vi "Keithley_Output_to_Number_1_and_2.vi"(6 "GPIB = true, RS-232 = false":bool, 10 "string":string) -> (1 "number 2":dbl, 2 "number 1":dbl, 3 "array":dbl[](array[numeric]))   [LabVIEW 2018]
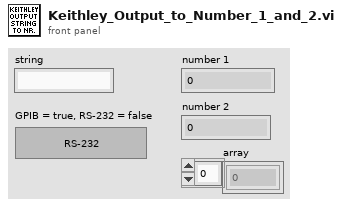
[diagram p1: front panel]
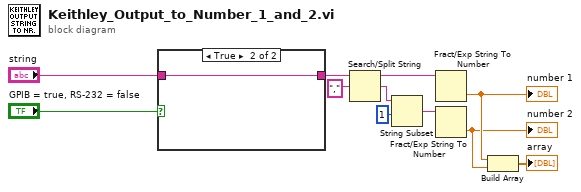
[diagram p0: block diagram]
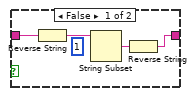
[diagram p2: hidden frame]
diagram:
  n1 = case shown="True" "GPIB = true, RS-232 = false" {
    tunnel: "string" -> [w13 w16]
    tunnel: [w12 w16] -> w2
    frame False {
      (unwired) 1
      n2 = Reverse String(1:w13) -> (0:w15:string)
      n3 = String Subset(string=w15) -> (substring=w14:string)  [unwired: 2 in]
      n4 = Reverse String(1:w14) -> (0:w12:string)
    }
    frame True {
    }
  }
  n5 = Search/Split String(string=w2, search string/char (-)=",") -> (substring before match=w7:string, match + rest of string=w10:string)  [unwired: 1 in, 1 out]
  n6 = String Subset(string=w10, offset (0)=1) -> (substring=w11:string)  [unwired: 1 in]
  n7 = Fract/Exp String To Number(string=w7) -> (number=w6:dbl)  [unwired: 3 in, 1 out]
  "number 1" <- w6
  n8 = Fract/Exp String To Number(string=w11) -> (number=w5:dbl)  [unwired: 3 in, 1 out]
  "number 2" <- w5
  n9 = Build Array(w6, w5) -> (→"array":dbl[])
